vi "Create MetaData Element.vi"(6 "MetaData Parameters":T4, 7 "Channel Properties":T3, 8 "error in (no error)":errorcluster, 9 "Type":T1, 10 "Name":string, 11 "Refnum In":T2 format="%.0x") -> (0 "error out":errorcluster, 2 "Channel Refnum":T2 format="%.0x", 3 "Refnum Out":T2 format="%.0x")   [LabVIEW 2018, in "Instrument Addon Scripting API.lvlib"]
uses:
  Instrument Addon Scripting API.lvlib
  Addon/Addon Shared/Types/MetaData Parameters.ctl
  Addon/Addon Shared/Types/Protocol Data Type.ctl
  Addon/Addon Shared/Types/Metadata Channel Type.ctl
  Addon/Addon Shared/Types/Type Cast Type.ctl
  Addon/Addon Shared/Types/Endian.ctl
  <vilib>/NI Veristand/Custom Device API/Custom Device Item Ref.ctl
  Channel Properties.ctl
  MetaData Channel Type.ctl
  <vilib>/NI Veristand/Custom Device API/Custom Device Channel.ctl
  <vilib>/NI Veristand/Custom Device API/Custom Device Channel Type.ctl
  Addon/Addon Shared/Types/FG Control.ctl
  Addon/Addon Shared/SubVIs/Constants.vi
  <vilib>/NI Veristand/Custom Device Tools/Custom Device Utility Library/NI VeriStand - Search for Item by GUID.vi
  <vilib>/NI Veristand/Custom Device API/NI VeriStand - Get Item Property.vi
  <vilib>/NI Veristand/Custom Device API/Get Item Property (U32).vi
  <vilib>/NI Veristand/Custom Device API/Get Item Property (String Array).vi
  <vilib>/NI Veristand/Custom Device API/Get Item Property (String).vi
  <vilib>/NI Veristand/Custom Device API/NI VeriStand - Set Item Property.vi
  <vilib>/NI Veristand/Custom Device API/Set Item Property (U32).vi
  <vilib>/NI Veristand/Custom Device API/Set Item Property (String Array).vi
  <vilib>/NI Veristand/Custom Device API/NI VeriStand - Get Item Children.vi
  <vilib>/NI Veristand/Custom Device API/NI VeriStand - Set Custom Device Channel Value Table.vi
  <vilib>/NI Veristand/Custom Device API/Set Item Property (String).vi
  <vilib>/NI Veristand/Custom Device Tools/Custom Device Utility Library/Custom Device Utility Library.lvlib
  Addon/Addon Shared/Instrument Addon Shared.lvlib
  <vilib>/NI Veristand/Custom Device API/Custom Device API.lvlib
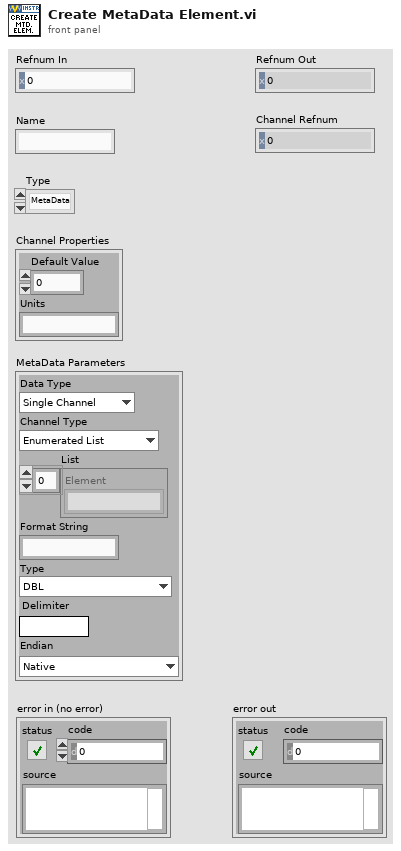
[diagram p1: front panel]
types:
  T1 = typedef "MetaData Channel Type.ctl" = enum16{"MetaData", "Global MetaData"}
  T2 = typedef "Custom Device API.lvlib/Custom Device Item Ref.ctl" = u64
  T3 = typedef "Channel Properties.ctl" = cluster{"Default Value":dbl, "Units":string}
  T4 = typedef "Instrument Addon Shared.lvlib/MetaData Parameters.ctl" = cluster{"Data Type":T5, "Channel Type":T6, "List":string[], "Format String":string, "Type":T7, "Delimiter":string, "Endian":T8}
  T5 = typedef "Instrument Addon Shared.lvlib/Protocol Data Type.ctl" = enum16{"Single Channel", "Array"}
  T6 = typedef "Instrument Addon Shared.lvlib/Metadata Channel Type.ctl" = enum16{"Enumerated List", "Format", "Type Cast"}
  T7 = typedef "Instrument Addon Shared.lvlib/Type Cast Type.ctl" = enum16{"DBL", "SGL", "U64", "U32", "U16", "U8", "I64", "I32", "I16", "I8"}
  T8 = typedef "Instrument Addon Shared.lvlib/Endian.ctl" = enum16{"Native", "Little", "Big"}
  T9 = typedef "Custom Device API.lvlib/Custom Device Channel Type.ctl" = enum16{"Input", "Output"}
  T10 = typedef "Instrument Addon Shared.lvlib/FG Control.ctl" = enum16{"Get", "Set"}
  T11 = typedef "Custom Device API.lvlib/Custom Device Channel.ctl" = cluster{"Type":T9, "Units":string, "Default Value":dbl, "Faultable":bool, "Scalable":bool}
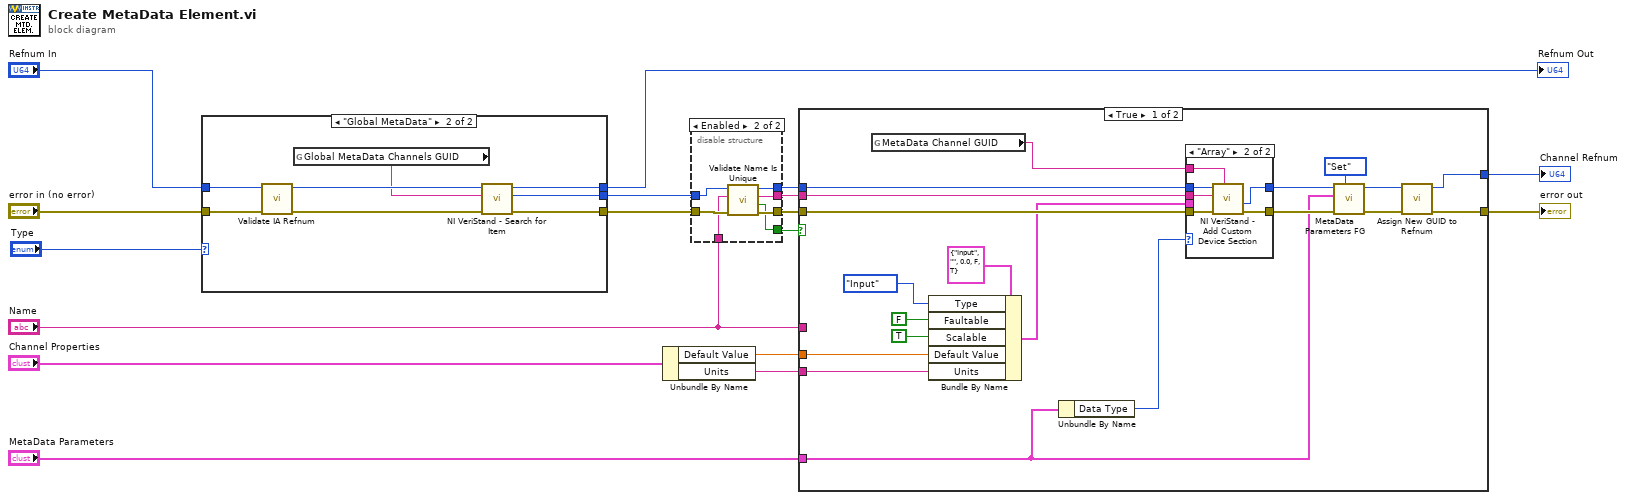
[diagram p0: block diagram]
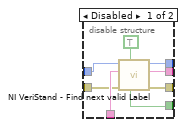
[diagram p2: hidden frame]
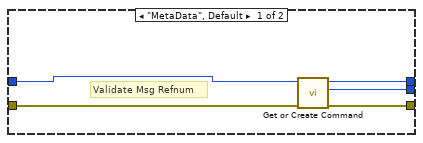
[diagram p3: hidden frame]
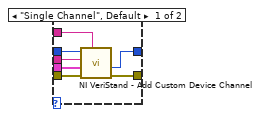
[diagram p4: hidden frame]
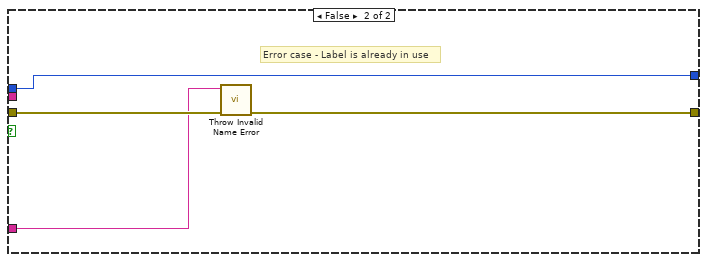
[diagram p5: hidden frame]
diagram:
  n1 = case shown="\"Global MetaData\"" "Type" {
    tunnel: [w19 w29] -> w9
    tunnel: [w22 w28] -> w8
    tunnel: "error in (no error)" -> [w21 w26]
    tunnel: "Refnum In" -> [w18 w24]
    tunnel: [w20 w23] -> w2
    frame "MetaData", Default {
      # "Validate Msg Refnum"
      n2 = call "Get or Create Command.vi"("error in (no error)"=w21, "Message Refnum In"=w18) -> ("error out"=w22:errorcluster, "Command Refnum"=w19:T2, "Message Refnum Out"=w20:T2)  [unwired: 7 in]
    }
    frame "Global MetaData" {
      n3 = call "Validate IA Refnum.vi"("Error In"=w26, "Refnum In"=w24) -> ("Error Out"=w27:errorcluster, "Refnum Out"=w30:T2)  [unwired: 7 in, 1 out]
      n4 = global read "Constants.vi" "Global MetaData Channels GUID"() -> (w25:string)
      n5 = call-poly <vilib>:"NI VeriStand - Search for Item.vi"("error in"=w27, "Item GUID"=w25, "Section Ref in"=w30) -> ("error out"=w28:errorcluster, "Item Ref"=w29:T2, "Section Ref out"=w23:T2)  [unwired: 5 in, 1 out]
    }
  }
  "Refnum Out" <- w2
  n6 = Unbundle By Name("Channel Properties") -> ("Default Value"=w5:dbl, "Units"=w4:string)
  n7 = disable-structure shown="Enabled" {
    disable-tunnel: "Name" -> [w38 w41]
    disable-tunnel: [w37 w39] -> w13
    disable-tunnel: [w36 w42] -> w12
    disable-tunnel: [w35 w43] -> w11
    disable-tunnel: [w34 w40] -> w10
    disable-tunnel: w9 -> [w32 w45]
    disable-tunnel: w8 -> [w31 w44]
    frame Disabled {
      n8 = call <vilib>:"NI VeriStand - Find next valid Label.vi"("Try requested Label only?"=TRUE, "error in (no error)"=w31, "Label"=w38, "Item Ref in"=w32) -> ("error out"=w35:errorcluster, "Label out"=w37:string, "Item Ref out"=w36:T2, "Requested label not in use?"=w34:bool)  [unwired: 3 in, 1 out]
    }
    frame Enabled {
      n9 = call "Validate Name Is Unique.vi"("error in (no error)"=w44, "Name in"=w41, "Parent Ref in"=w45) -> ("error out"=w43:errorcluster, "Unique?"=w40:bool, "Name out"=w39:string, "Parent Ref out"=w42:T2)  [unwired: 5 in]
    }
  }
  n10 = case shown="True" w10 {
    tunnel: w11 -> [w63 w81]
    tunnel: w12 -> [w65 w82]
    tunnel: w13 -> [w64 _]
    tunnel: [w58 w80] -> w14
    tunnel: [w56 w82] -> w15
    tunnel: "Name" -> [_ w79]
    tunnel: "MetaData Parameters" -> [w48 _]
    tunnel: w5 -> [w50 _]
    tunnel: w4 -> [w49 _]
    frame True {
      n11 = global read "Constants.vi" "MetaData Channel GUID"() -> (w46:string)
      n12 = Bundle By Name(cluster=T11 {"Type"=enum."Input", "Units"="", "Default Value"=0.0, "Faultable"=FALSE, "Scalable"=TRUE} ("Channel"), "Type"=Custom_Device_Channel_Type."Input", "Faultable"=FALSE, "Scalable"=TRUE, "Default Value"=w50, "Units"=w49) -> (w51:T11)
      n13 = Unbundle By Name(w48) -> ("Data Type"=w47:T5)
      n14 = case shown="\"Array\"" w47 {
        tunnel: w46 -> [w67 w74]
        tunnel: w65 -> [w72 w75]
        tunnel: w64 -> [w71 w73]
        tunnel: w63 -> [w70 w78]
        tunnel: [w69 w77] -> w61
        tunnel: [w66 w76] -> w60
        tunnel: w51 -> [w68 _]
        frame "Single Channel", Default {
          n15 = call <vilib>:"NI VeriStand - Add Custom Device Channel.vi"("GUID (Default Channel)"=w67, "error in (no error)"=w70, "Channel"=w68, "Channel Name"=w71, "Parent Ref in"=w72) -> ("error out"=w69:errorcluster, "Channel Ref"=w66:T2)  [unwired: 3 in, 2 out]
        }
        frame "Array" {
          n16 = call <vilib>:"NI VeriStand - Add Custom Device Section.vi"("GUID (Default Section)"=w74, "error in (no error)"=w78, "Section Name"=w73, "Parent Ref in"=w75) -> ("error out"=w77:errorcluster, "Section Ptr"=w76:T2)  [unwired: 4 in, 2 out]
        }
      }
      n17 = call "MetaData Parameters FG.vi"("Action"=FG_Control."Set", "error in (no error)"=w61, "MetaData Parameters"=w48, "Item Ref in"=w60) -> ("error out"=w59:errorcluster, "Item Ref out"=w57:T2)  [unwired: 5 in, 1 out]
      n18 = call "Assign New GUID to Refnum.vi"("error in (no error)"=w59, "Item Ref in"=w57) -> ("error out"=w58:errorcluster, "Item Ref out"=w56:T2)  [unwired: 8 in]
    }
    frame False {
      # "Error case - Label is already in use"
      n19 = call "Throw Invalid Name Error.vi"("error in (no error)"=w81, "Name"=w79) -> ("error out"=w80:errorcluster)  [unwired: 9 in]
    }
  }
  "Channel Refnum" <- w15
  "error out" <- w14
